vi "Team Name.vi"(11 "MyTeam in":refnum<class "MyTeam.lvclass">) -> (2 "Team Name":string)   [LabVIEW 2020, in "Galaxy.lvlib" / "MyTeam.lvclass"]
uses:
  MyTeam.lvclass
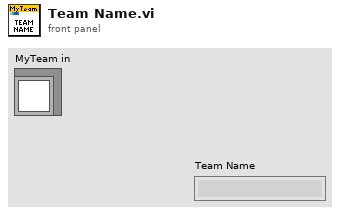
[diagram p1: front panel]
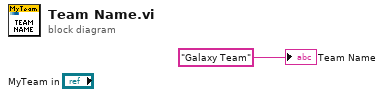
[diagram p0: block diagram]
diagram:
  "Team Name" <- "Galaxy Team" ("Team Name")
